vi "Read_Globe_Var.vi"() -> (3 "Global_Var":T1)   [LabVIEW 2014]
uses:
  General_VI/Global Var.vi
panel:
  out "Infeed_Joystick_Map":cluster{"X_Array":dbl[], "Y_Array":dbl[]}(graph)
  in  "Eject_X_Array":dbl[](array[numeric])=[-1.0, -0.2, 0.0, 0.2, 1.0, 0.0, 0.0, 0.0, 0.0, 0.0, 100.0]
  in  "Eject_Y_Array":dbl[](array[numeric])=[-1.0, 0.0, 0.0, 0.0, 1.0]
  in  "Ele_Y_Array":dbl[](array[numeric])=[-1.0, 0.0, 0.0, 0.0, 1.0]
  in  "Ele_X_Array":dbl[](array[numeric])=[-1.0, -0.2, 0.0, 0.2, 1.0, 0.0, 0.0, 0.0, 0.0, 0.0, 100.0]
  out "Eject_Joystick_Map":cluster{"X_Array":dbl[], "Y_Array":dbl[]}(graph)
  # "Reads all global joystick varibles"
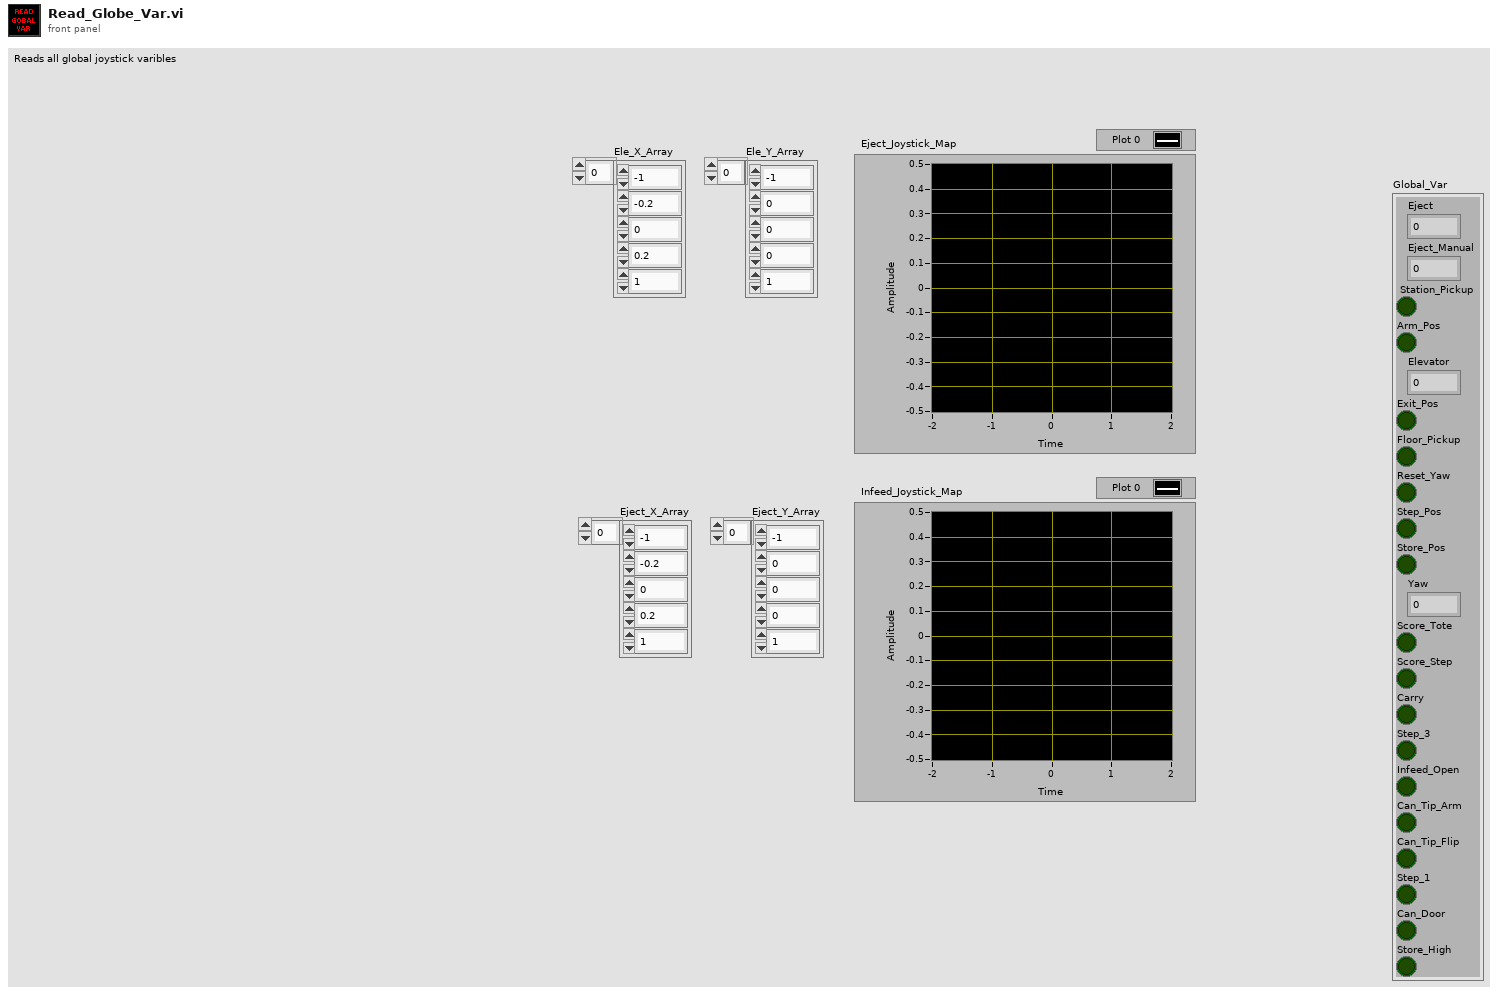
[diagram p1: front panel]
types:
  T1 = cluster{"Eject":dbl, "Eject_Manual":dbl, " Station_Pickup":bool, "Arm_Pos":bool, "Elevator":dbl, "Exit_Pos":bool, "Floor_Pickup":bool, "Reset_Yaw":bool, "Step_Pos":bool, "Store_Pos":bool, "Yaw":dbl, "Score_Tote":bool, "Score_Step":bool, "Carry":bool, "Step_3":bool, "Infeed_Open":bool, "Can_Tip_Arm":bool, "Can_Tip_Flip":bool, "Step_1":bool, "Can_Door":bool, "Store_High":bool}
  T2 = cluster{"Eject_X_Array":dbl[], "Eject_Y_Array":dbl[]}
  T3 = cluster{"Ele_X_Array":dbl[], "Ele_Y_Array":dbl[]}
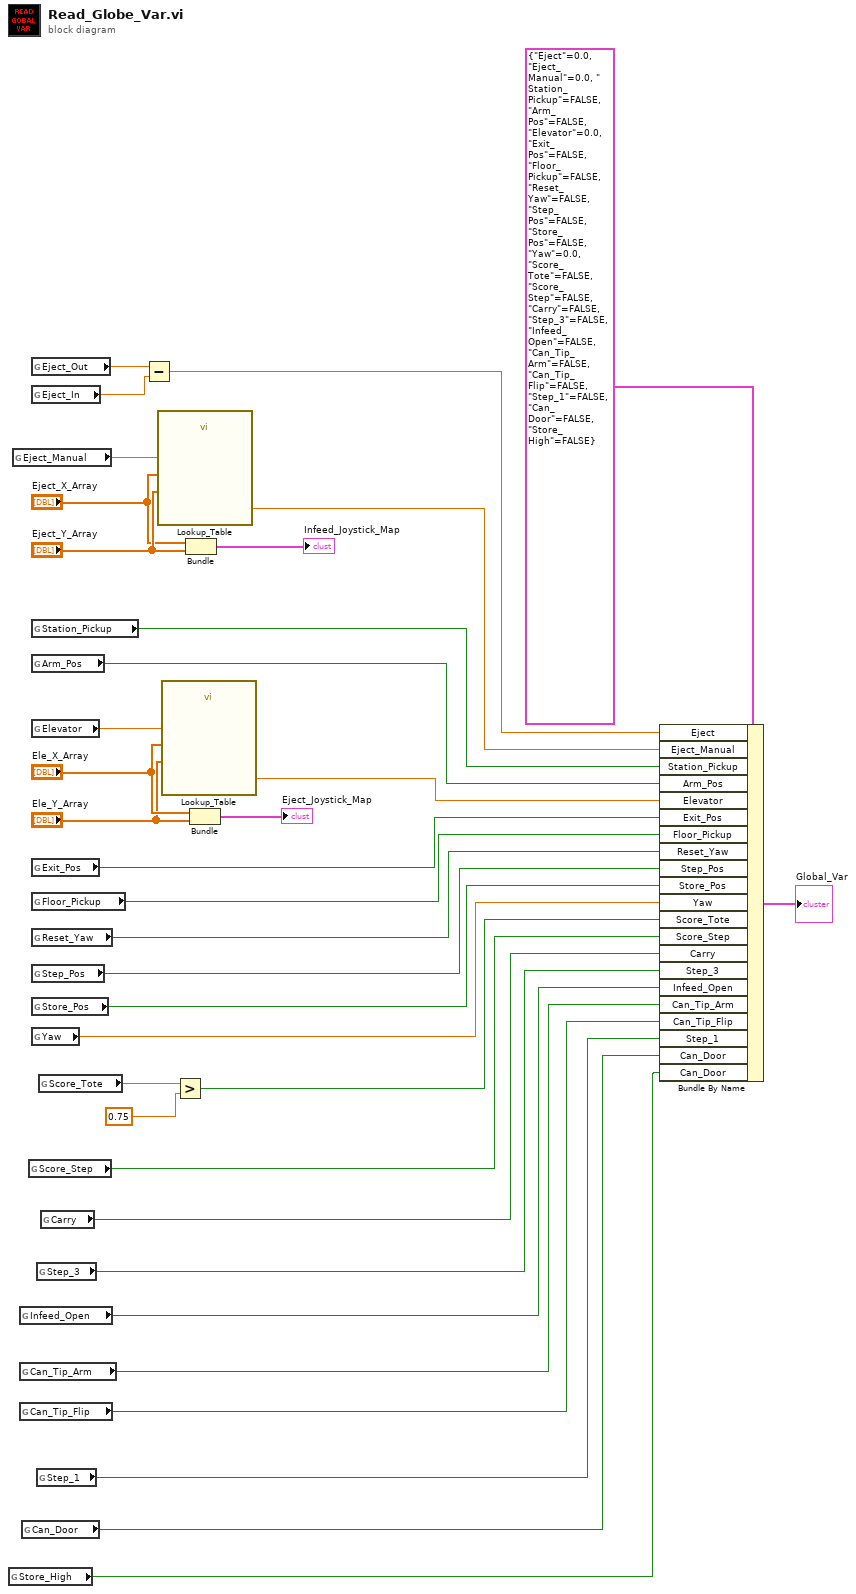
[diagram p0: block diagram]
diagram:
  n1 = global read "Global Var.vi" "Store_High"() -> (w2:bool)
  n2 = global read "Global Var.vi" "Eject_Manual"() -> (w24:dbl)
  n3 = global read "Global Var.vi" "Infeed_Open"() -> (w8:bool)
  n4 = global read "Global Var.vi" "Can_Tip_Arm"() -> (w6:bool)
  n5 = global read "Global Var.vi" "Can_Tip_Flip"() -> (w5:bool)
  n6 = global read "Global Var.vi" "Can_Door"() -> (w3:bool)
  n7 = global read "Global Var.vi" "Score_Step"() -> (w11:bool)
  n8 = global read "Global Var.vi" "Eject_Out"() -> (w29:dbl)
  n9 = global read "Global Var.vi" "Eject_In"() -> (w28:dbl)
  n10 = global read "Global Var.vi" "Station_Pickup"() -> (w26:bool)
  n11 = global read "Global Var.vi" "Arm_Pos"() -> (w25:bool)
  n12 = global read "Global Var.vi" "Elevator"() -> (w22:dbl)
  n13 = global read "Global Var.vi" "Exit_Pos"() -> (w20:bool)
  n14 = global read "Global Var.vi" "Floor_Pickup"() -> (w19:bool)
  n15 = global read "Global Var.vi" "Reset_Yaw"() -> (w18:bool)
  n16 = global read "Global Var.vi" "Step_Pos"() -> (w17:bool)
  n17 = global read "Global Var.vi" "Store_Pos"() -> (w16:bool)
  n18 = global read "Global Var.vi" "Yaw"() -> (w15:dbl)
  n19 = global read "Global Var.vi" "Step_3"() -> (w9:bool)
  n20 = global read "Global Var.vi" "Step_1"() -> (w4:bool)
  n21 = global read "Global Var.vi" "Score_Tote"() -> (w14:dbl)
  n22 = global read "Global Var.vi" "Carry"() -> (w10:bool)
  n23 = Subtract(x=w29, y=w28) -> (x-y=w27:dbl)
  n24 = call "Lookup_Table.vi"("Y_Array"="Eject_Y_Array", "x_in"=w24, "X_Array"="Eject_X_Array") -> ("y_out"=w23:dbl)  [unwired: 6 in]
  n25 = call "Lookup_Table.vi"("Y_Array"="Ele_Y_Array", "x_in"=w22, "X_Array"="Ele_X_Array") -> ("y_out"=w21:dbl)  [unwired: 6 in]
  n26 = Greater?(x=w14, y=0.75) -> (0:w12:bool)
  n27 = Bundle("Eject_X_Array"="Eject_X_Array", "Eject_Y_Array"="Eject_Y_Array") -> (→"Infeed_Joystick_Map":T2)  [unwired: 1 in]
  n28 = Bundle("Ele_X_Array"="Ele_X_Array", "Ele_Y_Array"="Ele_Y_Array") -> (→"Eject_Joystick_Map":T3)  [unwired: 1 in]
  n29 = Bundle By Name(cluster=T1 {"Eject"=0.0, "Eject_Manual"=0.0, " Station_Pickup"=FALSE, "Arm_Pos"=FALSE, "Elevator"=0.0, "Exit_Pos"=FALSE, "Floor_Pickup"=FALSE, "Reset_Yaw"=FALSE, "Step_Pos"=FALSE, "Store_Pos"=FALSE, "Yaw"=0.0, "Score_Tote"=FALSE, "Score_Step"=FALSE, "Carry"=FALSE, "Step_3"=FALSE, "Infeed_Open"=FALSE, "Can_Tip_Arm"=FALSE, "Can_Tip_Flip"=FALSE, "Step_1"=FALSE, "Can_Door"=FALSE, "Store_High"=FALSE}, "Eject"=w27, "Eject_Manual"=w23, "Station_Pickup"=w26, "Arm_Pos"=w25, "Elevator"=w21, "Exit_Pos"=w20, "Floor_Pickup"=w19, "Reset_Yaw"=w18, "Step_Pos"=w17, "Store_Pos"=w16, "Yaw"=w15, "Score_Tote"=w12, "Score_Step"=w11, "Carry"=w10, "Step_3"=w9, "Infeed_Open"=w8, "Can_Tip_Arm"=w6, "Can_Tip_Flip"=w5, "Step_1"=w4, "Can_Door"=w3, "Can_Door"=w2) -> (→"Global_Var":T1)
